vi "Start Sync.vi"(8 "error in (no error)":errorcluster, 11 "gRPC Server in":refnum<class "GreeterService.lvclass">) -> (0 "error out":errorcluster, 3 "gRPC Server out":refnum<class "GreeterService.lvclass">)   [LabVIEW 2019, in "Generated_server.lvlib" / "GreeterService.lvclass"]
uses:
  <vilib>/gRPC/gRPC Server and Client Template [2]/gRPC Scripting Tools/Generated_server/RPC Service/GreeterService/GreeterService.lvclass
panel:
  out "error out":errorcluster
  in  "error in":errorcluster
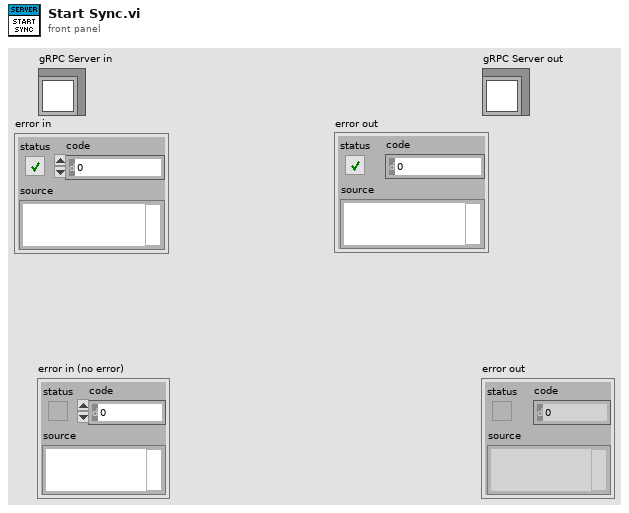
[diagram p1: front panel]
types:
  T1 = typedef "Generated_server.lvlib/GreeterService.lvclass/Server Internal UEs.ctl" = cluster{"GreeterService SayHello Internal UE":refnum<user-event>}
  T2 = typedef "Generated_server.lvlib/GreeterService.lvclass/Server gRPC UEs.ctl" = cluster{"GreeterService SayHello gRPC UE":refnum<user-event>}
  T3 = typedef "grpc-lvsupport-release.lvlib/grpcId.ctl" = u64
  T4 = typedef "Generated_server.lvlib/helloworld_HelloRequest.ctl" = cluster{"name":string}
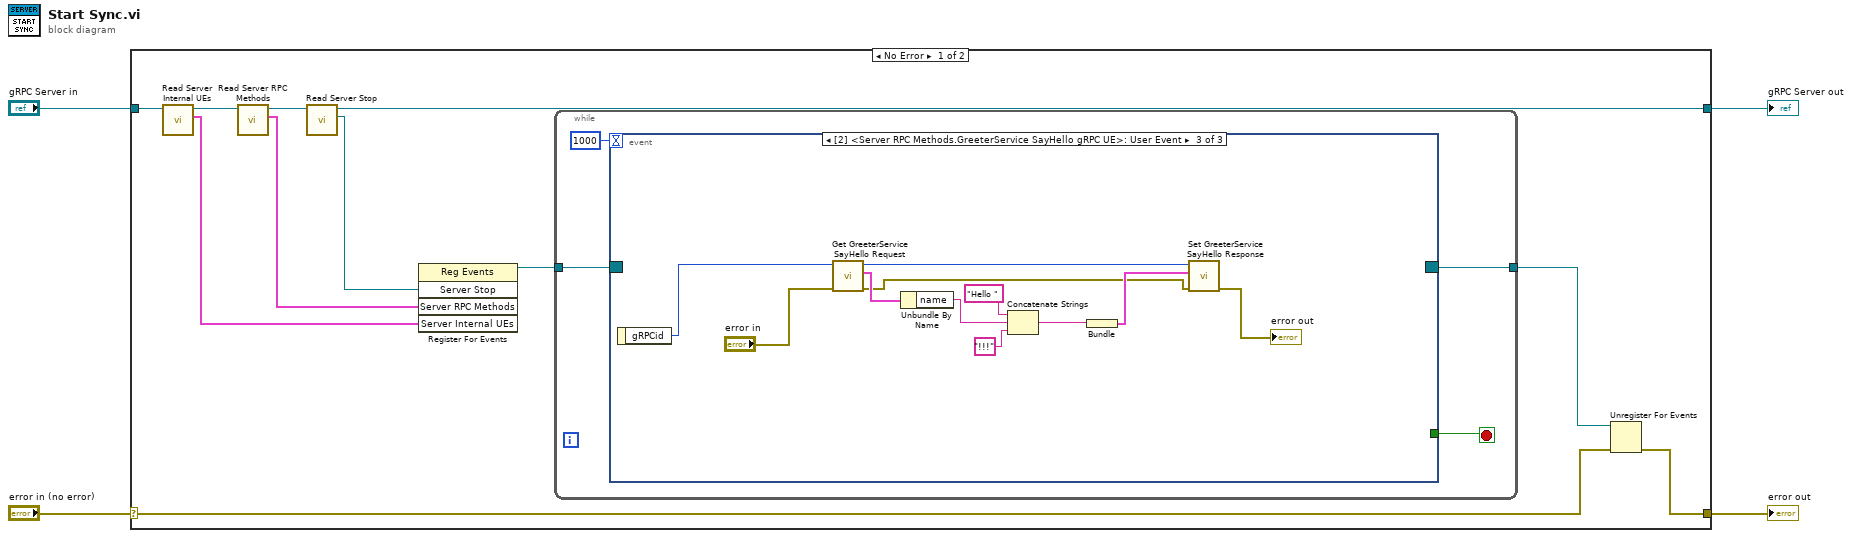
[diagram p0: block diagram]
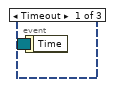
[diagram p2: hidden frame]
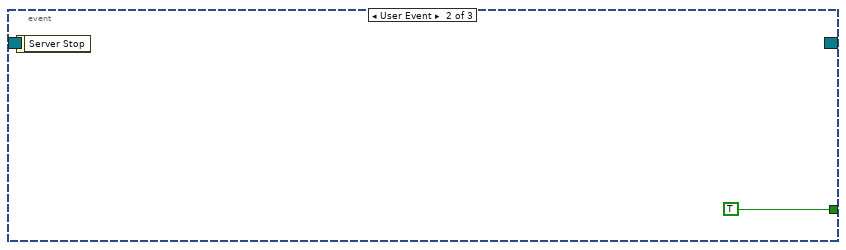
[diagram p3: hidden frame]
diagram:
  n1 = case shown="No Error" "error in (no error)" {
    selector: "error in (no error)" -> [w9 w33]
    tunnel: [w8 w33] -> w3
    tunnel: [w6 w32] -> w1
    tunnel: "gRPC Server in" -> [w15 w32]
    frame No Error {
      n2 = call <vilib>:"Read Server Internal UEs.vi"("gRPC service in"=w15) -> ("Server Internal UEs"=w13:T1, "gRPC service out"=w14:refnum<class "GreeterService.lvclass">)  [unwired: 8 in, 1 out]
      n3 = call <vilib>:"Read Server RPC Methods.vi"("gRPC service in"=w14) -> ("Server RPC Methods"=w7:T2, "gRPC service out"=w12:refnum<class "GreeterService.lvclass">)  [unwired: 8 in, 1 out]
      n4 = call-dynamic "Read Server Stop.vi"("gRPC service in"=w12) -> ("Server Stop"=w5:refnum<user-event>, "gRPC service out"=w6:refnum<class "GreeterService.lvclass">)  [unwired: 8 in, 1 out]
      n5 = register-events(w5, w7, w13) -> (reference out=w11:refnum<event-registration>)  [unwired: 2 in, 1 out]
      n6 = while {
        tunnel: w11 -> [w19]
        tunnel: [w17] -> w10
        stop <- w18 stop-if-true
        n7 = event "RPC Methods Event Structure" shown="[2] <Server RPC Methods.GreeterService SayHello gRPC UE>: User Event" {
          selector: w19 -> [_ _ _]
          dyn-events: [_ _ _] -> w17
          timeout: 1000 -> [_ _ _]
          tunnel: [_ TRUE _] -> w18
          event Timeout {
            n8 = event-data() -> ()  [unwired: 1 in, 1 out]
          }
          event User Event {
            n9 = event-data() -> ()  [unwired: 1 in, 1 out]
          }
          event User Event {
            n10 = event-data() -> ("gRPCid"=w31:T3)  [unwired: 1 in]
            n11 = call <vilib>:"Get GreeterService SayHello Request.vi"("error in (no error)"="error in", "gRPCid"=w31) -> ("error out"=w23:errorcluster, "Message Data"=w29:T4, "gRPCid out"=w30:T3)  [unwired: 7 in]
            n12 = Unbundle By Name(w29) -> ("name"=w28:string)
            n13 = Concatenate Strings("Hello " ("string"), w28, "!!!" ("string")) -> (w25:string)
            n14 = Bundle(w25) -> (w24:cluster{string})  [unwired: 1 in]
            n15 = call <vilib>:"Set GreeterService SayHello Response.vi"("error in (no error)"=w23, "Message Data"=w24, "gRPCid in"=w30) -> ("error out"=→"error out":errorcluster)  [unwired: 8 in]
          }
        }
      }
      n16 = Unregister For Events(event registration refnum=w10, error in=w9) -> (error out=w8:errorcluster)
    }
    frame Error {
    }
  }
  "error out" <- w3
  "gRPC Server out" <- w1
